vi "Step Counter.Inc Data_Info Level.vi"(1 "Step State":T1) -> (0 "Step State Out":T1)   [LabVIEW 2018]
uses:
  Step Counter.State Info.ctl
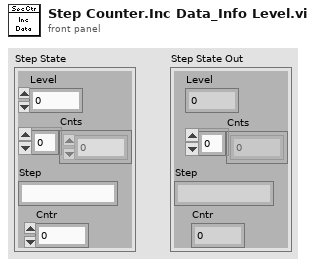
[diagram p1: front panel]
types:
  T1 = typedef "Step Counter.State Info.ctl" = cluster{"Level":i32, "Cnts":i32[], "Step":string, "Cntr":i32}
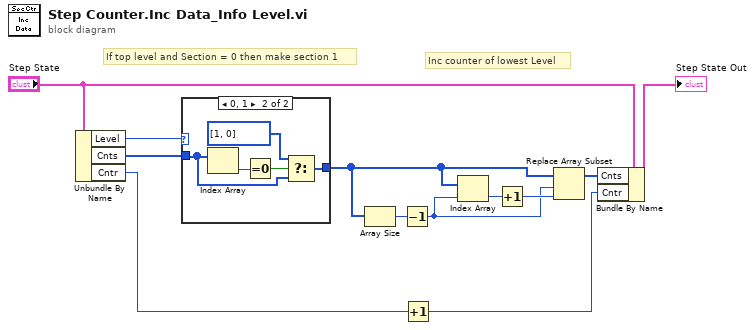
[diagram p0: block diagram]
diagram:
  # "Inc counter of lowest Level"
  # "If top level and Section = 0 then make section 1"
  n1 = Unbundle By Name("Step State") -> ("Level"=w7:i32, "Cnts"=w6:i32[], "Cntr"=w2:i32)
  n2 = case shown="0, 1" w7 {
    tunnel: w6 -> [w13 w15]
    tunnel: [w13 w16] -> w5
    frame Default {
    }
    frame 0, 1 {
      n3 = Index Array(array=w15) -> (element=w18:i32)  [unwired: 1 in]
      n4 = Equal To 0?(x=w18) -> (x = 0?=w17:bool)
      n5 = Select(t=i32[] [1, 0] ("Cnts"), s=w17, f=w15) -> (s? t:f=w16:i32[])
    }
  }
  n6 = Array Size(array=w5) -> (size(s)=w12:i32)
  n7 = Decrement(x=w12) -> (x-1=w9:i32)
  n8 = Increment(x=w2) -> (x+1=w1:i32)
  n9 = Index Array(array=w5, index=w9) -> (element=w11:i32)
  n10 = Increment(x=w11) -> (x+1=w10:i32)
  n11 = Replace Array Subset(array=w5, new element=w10, index=w9) -> (w8:i32[])
  n12 = Bundle By Name(cluster="Step State", "Cnts"=w8, "Cntr"=w1) -> (→"Step State Out":T1)
